vi "(SubVI)_2Ddisplay_BD_test.vi"(0 "data":dbl[][](array[numeric]), 1 "Image Avg 2D":dbl, 2 "Doppler 2D":bool, 5 "zero array":dbl[][](array[numeric]), 7 "first row":dbl[](array[numeric]), 9 "input cluster 3":T1, 11 "# of Cores":i32=3, 12 "Power 2D":dbl, 13 "Period":dbl) -> (4 "Image":dbl[][](array[numeric]), 6 "buffer out":dbl[][](array[numeric]), 8 "Image 2":dbl[](array[numeric]), 10 "velocity_profile":dbl[][](array[numeric]), 15 "error out":errorcluster)   [LabVIEW 2019]
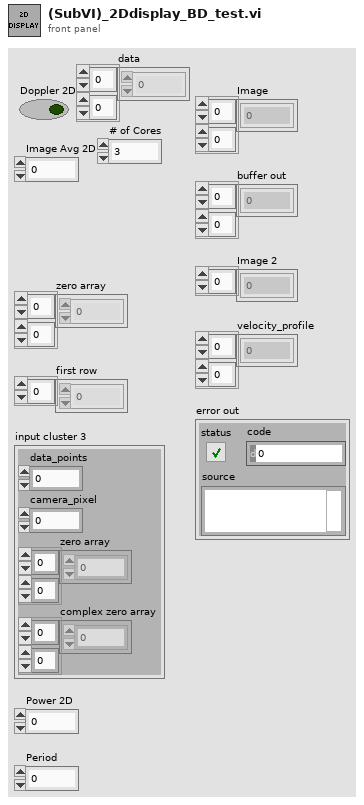
[diagram p1: front panel]
types:
  T1 = cluster{"data_points":i32, "camera_pixel":i32, "zero array":dbl[][], "complex zero array":dbl[][]}
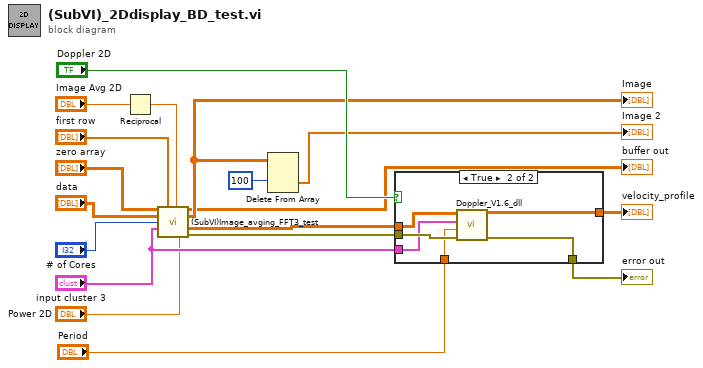
[diagram p0: block diagram]
diagram:
  n1 = Reciprocal(x="Image Avg 2D") -> (1/x=w10:dbl)
  n2 = call "(SubVI)Image_avging_FFT3_test.vi"("buffer in"="zero array", "index"="first row", "Average"=w10, "data"="data", "# of Cores"="# of Cores", "input cluster"="input cluster 3", "power"="Power 2D") -> ("buffer out"=→"buffer out":dbl[][], "Image"=w3:dbl[][], "complex_depth_profile"=w4:dbl[][], "error out"=w5:errorcluster)  [unwired: 5 in]
  "Image" <- w3
  n3 = Delete From Array(array=w3, index (row)=100 ("FT Index")) -> (deleted portion=→"Image 2":dbl[])  [unwired: 2 in, 1 out]
  n4 = case shown="True" "Doppler 2D" {
    tunnel: "input cluster 3" -> [_ w22]
    tunnel: w5 -> [w20 w26]
    tunnel: [w20 w25] -> w13
    tunnel: w4 -> [w19 w24]
    tunnel: "Period" -> [_ w23]
    tunnel: [w19 w21] -> w15
    frame False {
    }
    frame True {
      n5 = call "Doppler_V1.6_dll.vi"("error in (no error)"=w26, "period"=w23, "input cluster"=w22, "Data_complex"=w24) -> ("error out"=w25:errorcluster, "velocity_profile"=w21:dbl[][])  [unwired: 6 in]
    }
  }
  "velocity_profile" <- w15
  "error out" <- w13
